vi "WLF4_Setpointa.vi"(3 "error in (no error)":errorcluster, 4 "Set Point 1":dbl, 5 "Instrument Resource Name":refnum<visa-resource-name>) -> (1 "Measured Temp":dbl)   [LabVIEW 2012]
doc: "This VI sets the system parameters which define the global operating characteristics of the controller.\n\nNote: It represents the <B>Main>Setup>System</B> menu of the controller."
panel:
  out "error out":errorcluster
  in  "Unit Address (1)":u8=1
  # "WATLOW F4 Series"
  # "Main > Setup > System Parameters"
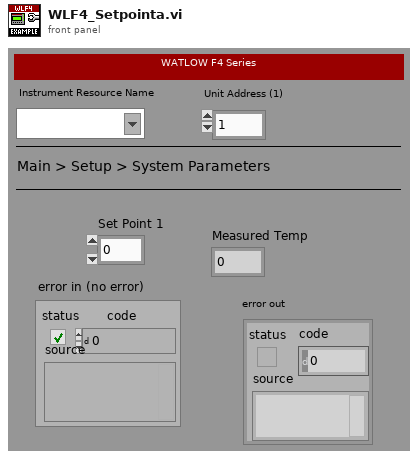
[diagram p1: front panel]
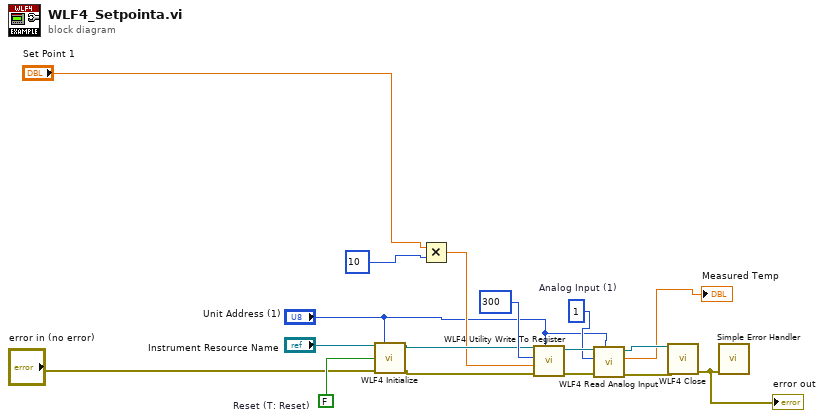
[diagram p0: block diagram]
diagram:
  w5 = i16 1  # Analog Input (1)
  w16 = FALSE  # Reset (T: Reset)
  n1 = call <instrlib>:"WLF4 Initialize.vi"("Instrument Resource Name"="Instrument Resource Name", "Unit Address (1)"="Unit Address (1)", "Reset (T: Reset)"=w16, "error in (no error)"="error in (no error)") -> ("dup VISA session"=w14:refnum<visa-resource-name>, "error out"=w13:errorcluster)  [unwired: 10 in]
  n2 = Multiply(x="Set Point 1", y=10) -> (x*y=w10:dbl)
  n3 = call <instrlib>:"WLF4 Utility Write To Register.vi"("Unit Address (1)"="Unit Address (1)", "error in (no error)"=w13, "Data (0)"=w10, "Register Address (0)"=300, "VISA session"=w14) -> ("error out"=w8:errorcluster, "dup VISA session"=w9:refnum<visa-resource-name>)  [unwired: 5 in]
  n4 = call <instrlib>:"WLF4 Read Analog Input.vi"("Unit Address (1)"="Unit Address (1)", "error in (no error)"=w8, "Analog Input (1)"=w5, "VISA session"=w9) -> ("error out"=w7:errorcluster, "Value"=→"Measured Temp":dbl, "dup VISA session"=w6:refnum<visa-resource-name>)  [unwired: 5 in]
  n5 = call <instrlib>:"WLF4 Close.vi"("VISA session"=w6, "error in (no error)"=w7) -> ("error out"=w1:errorcluster)  [unwired: 13 in]
  "error out" <- w1
  n6 = call <vilib>:"Simple Error Handler.vi"("error in (no error)"=w1) -> ()  [unwired: 4 in, 5 out]
